vi "PH_Sequencer.PC PSDB Info.vi"(0 "i ref in":refnum<vi>, 1 "data":i8[](array[numeric]), 2 "Service Name":string, 3 "no link":bool, 4 "typeDescriptor":string, 5 "error IO":errorcluster) -> (14 "i ref out":refnum<vi>, 19 "error out":errorcluster)   [LabVIEW 2014, in "PH_Sequencer.lvlib"]
doc: "This VI gets the PSDB Information."
uses:
  PH_Sequencer.lvlib
  PH_Basics/PH_Common/PH_Common.lvlib
  CS_Core/CSSystem/CoreLib/CoreLib.lvlib
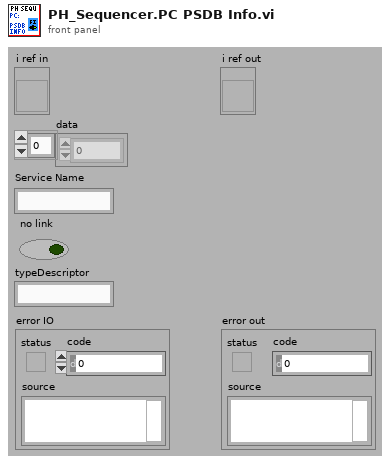
[diagram p1: front panel]
types:
  T1 = typedef "PH_Sequencer.lvlib/PH_Sequencer.i attribute.ctl" = cluster{"GUI Refs":cluster{"Main Off":refnum<vi>, "Fire":refnum<vi>, "Status":refnum<vi>, "Ready":refnum<vi>, "Waiting Time":refnum<vi>, "Timeout":refnum<vi>, "PPMA Ready":refnum<vi>, "Sequencer SM State":refnum<vi>, "PPPA Ready":refnum<vi>, "Calorimeter":refnum<vi>, "Beamline Ready":refnum<vi>, "Clear Beamline":refnum<vi>, "Linkage PPMA Rods":refnum<vi>, "Linkage Current PA":refnum<vi>, "Linkage Current MA":refnum<vi>, "Timing Ready":refnum<vi>, "State Timing":refnum<vi>, "Force Timing":refnum<vi>, "PSDB Shot Comment":refnum<vi>, "State PA Backreflection":refnum<vi>, "Beamline Z6 Ready":refnum<vi>, "Clear Z6 Beamline":refnum<vi>, "Sequence length":refnum<vi>, "Timing Mode":refnum<vi>, "Slow Trigger Settings":refnum<vi>, "Experiment Description":refnum<vi>, "State PSDB":refnum<vi>, "PSDB Ready":refnum<vi>, "Set PSDB Settings":refnum<vi>, "Get PSDB Info":refnum<vi>, "Take Snapshot":refnum<vi>, "Shottype":refnum<vi>, "Experiment":refnum<vi>, "Phase Frontends":refnum<vi>, "PP 45mm PILC in use":refnum<vi>}, "Status Info":cluster{"Machine Status":T2, "WaitingTime":i32, "Timeout":bool}, "Readyness":cluster{"Ready to shot":bool, "PPMA Ready":bool, "PPPA Ready":bool, "BL Ready":bool, "Timing Ready":bool, "BL Z6 Ready":bool, "PSDBReady":bool}, "Instancenames":cluster{"PPMA Rods":string, "PP Current Meas":string, "PH Beamline Chief":string, "PA Backrefl Meas":string, "Z6 Beamline Chief":string}, "Data to read":bool, "Calorimeter":cluster{"Instancename":string, "On":bool, "linked":bool}, "Linkage":cluster{"PPMA Rods":bool, "PP Current Meas":bool, "PHELIX Beamline Chief":bool, "PA Backrefl Meas":bool, "Z6 Beamline Chief":bool}, "Timing":cluster{"Instance":string, "linked":bool, "Status":T2, "Timing Mode":T3, "Slow Trigger Settings":T4, "Info available":cluster{"ext SlowTrigger":bool, "T2":bool, "Mode":bool, "Delay Slow Trigger":bool, "Phase FEs":bool}, "FE Phase":T5}, "Service ID R2S":i32, "PSDB":cluster{"Controller Instance":string, "Controller Status":T2, "Controller linked":bool, "Settings acknowledged":bool, "Current Experiment ID":i16, "Current Shot Type":i16, "Current Comment":string, "Remember Settings":bool, "Write 2 early":bool}, "PSDB Data":cluster{"Main Off?":bool, "Sequence Length":dbl, "Sequence startet":timestamp}, "6P 4Q Positions":cluster{"Instancename":string, "linked":bool, "Position":T6}[], "PUs":T7[]}
  T2 = typedef "PH_StatusHandler.lvlib/PH_StatusHandler.Status.ctl" = i16
  T3 = typedef "PH_Timing.lvlib/PH_Timing.Timing Mode.ctl" = cluster{"T2":i16, "Modeselector":enum32{"10 Hz", "0.5 Hz", "Shot"}}
  T4 = typedef "PH_Timing.lvlib/PH_Timing.Slow Trigger Settings.ctl" = cluster{"Delay":dbl, "externally triggered?":bool}
  T5 = typedef "PH_Timing.lvlib/PH_Timing.Phase FEs.ctl" = cluster{"Phase":dbl}
  T6 = typedef "PH_4_Pos_Selector.lvlib/PH_4_Pos_Selector.Position Selector.ctl" = u16
  T7 = typedef "PH_Sequencer.lvlib/PH_Sequencer.Head.ctl" = cluster{"PowerUnit":T8, "GUI Ref":refnum<vi>, "Information":T9, "linked?":bool, "GUI Ref Current Voltage":refnum<vi>}
  T8 = typedef "PH_PP_Common.lvlib/PH_PP_Common.PUs.ctl" = enum16{"no Info", "PA-19mm-1", "PA-19mm-2", "PA-45mm-PILC", "PA-45mm-MAIN", "MA-PU-1", "MA-PU-2", "MA-PU-3", "MA-PU-4", "MA-PU-5", "MA-PU-6", "MA-FR", "MA-PILC", "PA-45mm-DP"}
  T9 = typedef "PH_Sequencer.lvlib/PH_Sequencer.PU Information.ctl" = cluster{"State":T2, "Waiting Time [s]":dbl, "PU State SM":T10, "PU Timeout SM":T10}
  T10 = typedef "PH_PowerUnit_BaseClass.lvlib/PH_PowerUnit_BaseClass.SM States.ctl" = enum16{".", "Stand by", "Switch PU on", "Configure", "Set Default Voltage", "Set STANDBY", "Set READY", "Wait for Shot Cmd", "Open Dump Rods", "Open Ross Relais", "Close Ross Relais", "Switch PSU on", "Switch PSU off", "Charge", "Switch GD Channel on", "Close Dump Rods", "Rods-TO", "RR-TO", "PSU-TO", "Trigger-TO"}
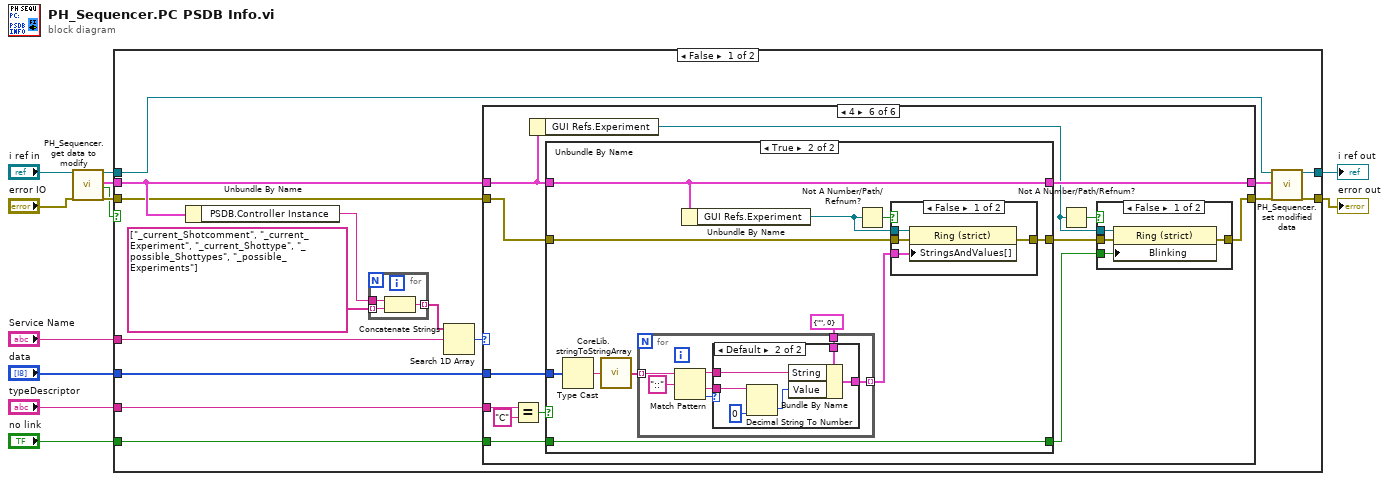
[diagram p0: block diagram]
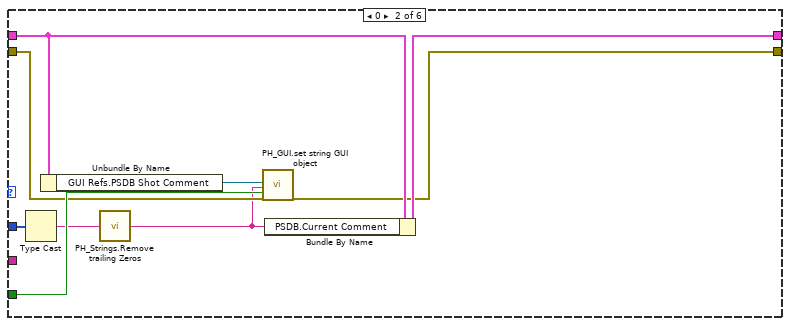
[diagram p3: hidden frame]
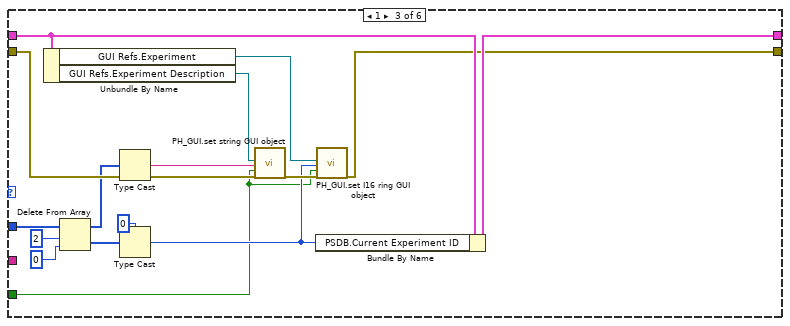
[diagram p4: hidden frame]
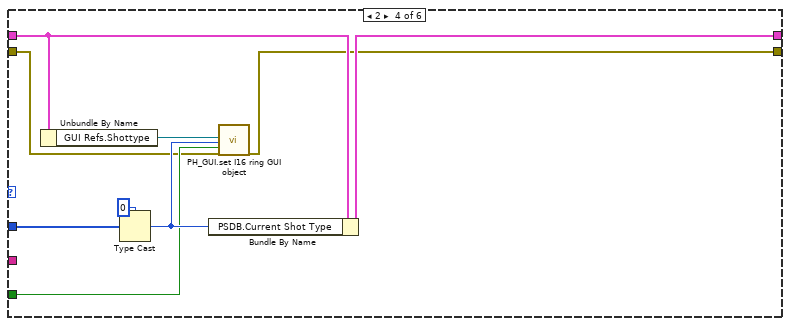
[diagram p5: hidden frame]
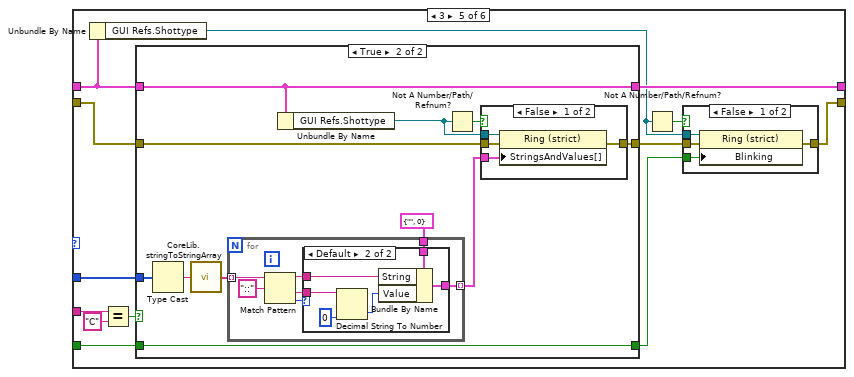
[diagram p6: hidden frame]
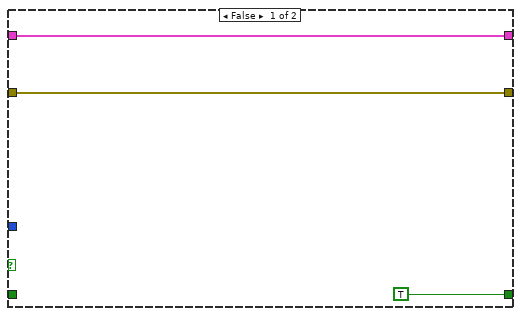
[diagram p7: hidden frame]
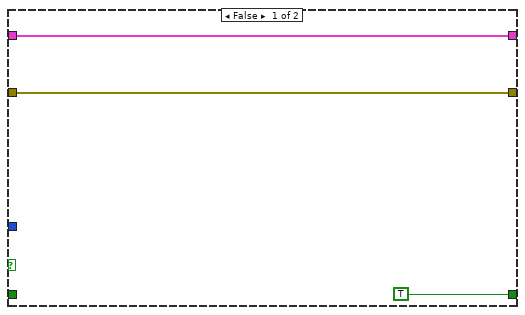
[diagram p11: hidden frame]
diagram:
  n1 = call "PH_Sequencer.get data to modify.vi"("i ref in"="i ref in", "error in (no error)"="error IO") -> ("i ref out"=w8:refnum<vi>, "i attribute"=w12:T1, "timed out"=w4:bool, "error out"=w7:errorcluster)  [unwired: 14 in]
  n2 = case shown="False" w4 {
    tunnel: w12 -> [w19 _]
    tunnel: "Service Name" -> [w24 _]
    tunnel: w8 -> [w14 w170]
    tunnel: w7 -> [w17 w169]
    tunnel: [w23 w169] -> w6
    tunnel: [w22 w170] -> w5
    tunnel: "no link" -> [w18 _]
    tunnel: "data" -> [w15 _]
    tunnel: "typeDescriptor" -> [w13 _]
    frame False {
      n3 = Unbundle By Name(w19) -> ("PSDB.Controller Instance"=w27:string)
      n4 = for {
        tunnel: w27 -> [w168]
        tunnel: string[] ["_current_Shotcomment", "_current_Experiment", "_current_Shottype", "_possible_Shottypes", "_possible_Experiments"] -> [w167] mode=indexing
        tunnel: [w166] -> w25 mode=indexing
        n5 = Concatenate Strings(w168, w167) -> (w166:string)
      }
      n6 = Search 1D Array(1D array=w25, element=w24) -> (index of element=w21:i32)  [unwired: 1 in]
      n7 = case shown="4" w21 {
        tunnel: [w29 w38 w54 w63 w76 w127] -> w20
        tunnel: w19 -> [w29 w37 w53 w60 w71 w122]
        tunnel: w18 -> [_ w35 w39 w57 w67 w118]
        tunnel: w17 -> [w28 w33 w46 w56 w75 w126]
        tunnel: [w28 w34 w41 w55 w72 w123] -> w16
        tunnel: w15 -> [_ w32 w48 w61 w69 w120]
        tunnel: w13 -> [_ _ _ _ w66 w117]
        frame Default {
        }
        frame 0 {
          n8 = Type Cast(x=w32) -> (*(type *) &x=w31:string)  [unwired: 1 in]
          n9 = Unbundle By Name(w37) -> ("GUI Refs.PSDB Shot Comment"=w36:refnum<vi>)
          n10 = call "PH_Strings.Remove trailing Zeros.vi"("Input String"=w31) -> ("Output String"=w30:string)
          n11 = call "PH_GUI.set string GUI object.vi"("GUI object Ref"=w36, "Text"=w30, "Blinking? (false)"=w35, "error in"=w33) -> ("error out"=w34:errorcluster)  [unwired: 15 in]
          n12 = Bundle By Name(cluster=w37, "PSDB.Current Comment"=w30) -> (w38:T1)
        }
        frame 1 {
          n13 = Unbundle By Name(w53) -> ("GUI Refs.Experiment"=w43:refnum<vi>, "GUI Refs.Experiment Description"=w52:refnum<vi>)
          n14 = Delete From Array(array=w48, length=2, index=0) -> (deleted portion=w47:i8[], array with subset deleted=w45:i8[])
          n15 = Type Cast(x=w45) -> (*(type *) &x=w44:string)  [unwired: 1 in]
          n16 = Type Cast(type=i16 0, x=w47) -> (*(type *) &x=w40:i16)
          n17 = call "PH_GUI.set string GUI object.vi"("GUI object Ref"=w52, "Text"=w44, "Blinking? (false)"=w39, "error in"=w46) -> ("error out"=w42:errorcluster)  [unwired: 15 in]
          n18 = Bundle By Name(cluster=w53, "PSDB.Current Experiment ID"=w40) -> (w54:T1)
          n19 = call "PH_GUI.set I16 ring GUI object.vi"("Ring Ref"=w43, "Value"=w40, "Blinking (false)"=w39, "error in (no error)"=w42) -> ("error out"=w41:errorcluster)  [unwired: 15 in]
        }
        frame 2 {
          n20 = Unbundle By Name(w60) -> ("GUI Refs.Shottype"=w59:refnum<vi>)
          n21 = Type Cast(type=i16 0, x=w61) -> (*(type *) &x=w58:i16)
          n22 = Bundle By Name(cluster=w60, "PSDB.Current Shot Type"=w58) -> (w63:T1)
          n23 = call "PH_GUI.set I16 ring GUI object.vi"("Ring Ref"=w59, "Value"=w58, "Blinking (false)"=w57, "error in (no error)"=w56) -> ("error out"=w55:errorcluster)  [unwired: 15 in]
        }
        frame 3 {
          n24 = Unbundle By Name(w71) -> ("GUI Refs.Shottype"=w70:refnum<vi>)
          n25 = Equal?(x=w66, y="C") -> (x = y?=w64:bool)
          n26 = case shown="True" w64 {
            tunnel: [w79 w88] -> w76
            tunnel: w75 -> [w78 w90]
            tunnel: [w78 w89] -> w73
            tunnel: w71 -> [w79 w88]
            tunnel: w69 -> [_ w86]
            tunnel: [TRUE ("no link") w87] -> w68
            tunnel: w67 -> [_ w87]
            frame False {
            }
            frame True {
              n27 = Type Cast(x=w86) -> (*(type *) &x=w85:string)  [unwired: 1 in]
              n28 = call "CoreLib.stringToStringArray.vi"("String"=w85) -> ("Array"=w80:string[])
              n29 = for {
                tunnel: [w96] -> w82 mode=indexing
                tunnel: cluster{"String":string, "Value":i16} {"String"="", "Value"=0} -> [w97]
                tunnel: w80 -> [w94] mode=indexing
                n30 = Match Pattern(string=w94, regular expression="::") -> (before substring=w93:string, after substring=w92:string, offset past match=w91:i32)  [unwired: 1 in, 1 out]
                n31 = case shown="Default" w91 {
                  tunnel: w97 -> [w98 w104]
                  tunnel: [w98 w103] -> w96
                  tunnel: w93 -> [_ w102]
                  tunnel: w92 -> [_ w101]
                  frame -1 {
                  }
                  frame Default {
                    n32 = Decimal String To Number(string=w101, default (0L)=i16 0 ("Value")) -> (number=w99:i16)  [unwired: 1 in, 1 out]
                    n33 = Bundle By Name(cluster=w104, "String"=w102, "Value"=w99) -> (w103:cluster{"String":string, "Value":i16})
                  }
                }
              }
              n34 = Unbundle By Name(w88) -> ("GUI Refs.Shottype"=w83:refnum<vi>)
              n35 = Not A Number/Path/Refnum?(number/path/refnum=w83) -> (NaN/Path/Refnum?=w84:bool)
              n36 = case shown="False" w84 {
                tunnel: w90 -> [w108 w109]
                tunnel: [w107 w109] -> w89
                tunnel: w83 -> [w106 _]
                tunnel: w82 -> [w105 _]
                frame False {
                  n37 = property class="Ring (strict)"(reference=w106, error in=w108, "StringsAndValues[]"=w105) -> (error out=w107:errorcluster)  [unwired: 1 out]
                }
                frame True {
                }
              }
            }
          }
          n38 = Not A Number/Path/Refnum?(number/path/refnum=w70) -> (NaN/Path/Refnum?=w74:bool)
          n39 = case shown="False" w74 {
            tunnel: w73 -> [w113 w114]
            tunnel: [w112 w114] -> w72
            tunnel: w70 -> [w111 _]
            tunnel: w68 -> [w110 _]
            frame False {
              n40 = property class="Ring (strict)"(reference=w111, error in=w113, "Blinking"=w110) -> (error out=w112:errorcluster)  [unwired: 1 out]
            }
            frame True {
            }
          }
        }
        frame 4 {
          n41 = Equal?(x=w117, y="C") -> (x = y?=w115:bool)
          n42 = Unbundle By Name(w122) -> ("GUI Refs.Experiment"=w121:refnum<vi>)
          n43 = case shown="True" w115 {
            tunnel: [w130 w139] -> w127
            tunnel: w126 -> [w129 w141]
            tunnel: [w129 w140] -> w124
            tunnel: w122 -> [w130 w139]
            tunnel: w120 -> [_ w137]
            tunnel: [TRUE ("no link") w138] -> w119
            tunnel: w118 -> [_ w138]
            frame False {
            }
            frame True {
              n44 = Type Cast(x=w137) -> (*(type *) &x=w136:string)  [unwired: 1 in]
              n45 = call "CoreLib.stringToStringArray.vi"("String"=w136) -> ("Array"=w131:string[])
              n46 = for {
                tunnel: [w147] -> w133 mode=indexing
                tunnel: cluster{"String":string, "Value":i16} {"String"="", "Value"=0} -> [w148]
                tunnel: w131 -> [w145] mode=indexing
                n47 = Match Pattern(string=w145, regular expression="::") -> (before substring=w144:string, after substring=w143:string, offset past match=w142:i32)  [unwired: 1 in, 1 out]
                n48 = case shown="Default" w142 {
                  tunnel: w148 -> [w149 w155]
                  tunnel: [w149 w154] -> w147
                  tunnel: w144 -> [_ w153]
                  tunnel: w143 -> [_ w152]
                  frame -1 {
                  }
                  frame Default {
                    n49 = Decimal String To Number(string=w152, default (0L)=i16 0 ("Value")) -> (number=w150:i16)  [unwired: 1 in, 1 out]
                    n50 = Bundle By Name(cluster=w155, "String"=w153, "Value"=w150) -> (w154:cluster{"String":string, "Value":i16})
                  }
                }
              }
              n51 = Unbundle By Name(w139) -> ("GUI Refs.Experiment"=w134:refnum<vi>)
              n52 = Not A Number/Path/Refnum?(number/path/refnum=w134) -> (NaN/Path/Refnum?=w135:bool)
              n53 = case shown="False" w135 {
                tunnel: w141 -> [w159 w160]
                tunnel: [w158 w160] -> w140
                tunnel: w134 -> [w157 _]
                tunnel: w133 -> [w156 _]
                frame False {
                  n54 = property class="Ring (strict)"(reference=w157, error in=w159, "StringsAndValues[]"=w156) -> (error out=w158:errorcluster)  [unwired: 1 out]
                }
                frame True {
                }
              }
            }
          }
          n55 = Not A Number/Path/Refnum?(number/path/refnum=w121) -> (NaN/Path/Refnum?=w125:bool)
          n56 = case shown="False" w125 {
            tunnel: w124 -> [w164 w165]
            tunnel: [w163 w165] -> w123
            tunnel: w121 -> [w162 _]
            tunnel: w119 -> [w161 _]
            frame False {
              n57 = property class="Ring (strict)"(reference=w162, error in=w164, "Blinking"=w161) -> (error out=w163:errorcluster)  [unwired: 1 out]
            }
            frame True {
            }
          }
        }
      }
      n58 = call "PH_Sequencer.set modified data.vi"("i ref in"=w14, "i attribute"=w20, "error in (no error)"=w16) -> ("i ref out"=w22:refnum<vi>, "error out"=w23:errorcluster)  [unwired: 15 in]
    }
    frame True {
    }
  }
  "error out" <- w6
  "i ref out" <- w5
